vi "2 BoatInfotoStringSnapshot.vi"() -> (2 "Snapshot":string)   [LabVIEW 2011]
doc: "Makes a \"snapshot\" of robot status in string form, to be recorded in the log. Only notes what has changed since the last time."
uses:
  2 Classes/Waypoint/Waypoint.lvclass
  2 Globals/2 Global.vi
  Helper - Clean UTM Data.vi
  Helper - Clean Int Data.vi
  Helper - Clean String Data.vi
  Helper - Clean NoSail Data.vi
  Helper - Clean Boolean Data.vi
panel:
  in  "Array":string[](array[string])=["RobotLocation", "RobotHeading", "RobotVelocity", "RobotPitch", "RobotRoll", "BatteryVoltage", "ApparentWindDirection", "ApparentWindSpeed", "Rudder", "Sail", "GoodnessFunctions", "NoSailZones", "Waypoint#", "WaypointTolerance", "WaypointCoordinates", "OverrideRudder", "OverrideSail"]
  # "change this array if you want to record more things"
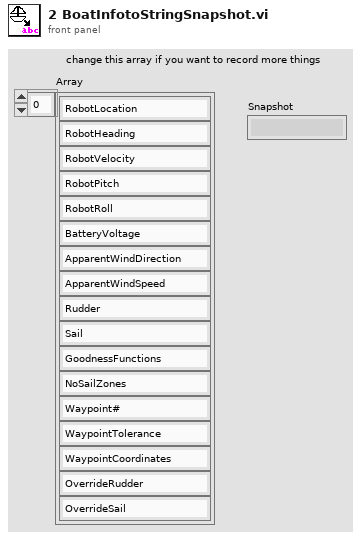
[diagram p1: front panel]
types:
  T1 = typedef "UTM Location.ctl" = cluster{"UTM Zone":dbl, "Hemisphere":enum16{"North", "South"}, "East":dbl, "North":dbl}
  T2 = typedef "heading.ctl" = dbl
  T3 = typedef "robot velocity.ctl" = cluster{"East":dbl, "North":dbl}
  T4 = typedef "pitch and roll.ctl" = cluster{"Pitch":dbl, "Roll":dbl}
  T5 = typedef "absolute wind direction.ctl" = dbl
  T6 = typedef "apparent wind speed.ctl" = dbl
  T7 = typedef "setpoints to boat.ctl" = cluster{"Sail Position":T8, "Rudder Angle":T9}
  T8 = typedef "sail setpt.ctl" = dbl
  T9 = typedef "rudder angle.ctl" = dbl
  T10 = typedef "Goodness Fns Indicator.ctl" = cluster{dbl, dbl, dbl[][]}
  T11 = typedef "UTM Circle.ctl" = cluster{"UTM Zone":dbl, "Hemisphere":enum16{"North", "South"}, "East":dbl, "North":dbl, "Radius":dbl}
  T12 = typedef "Current Waypoint.ctl" = i32
  T13 = typedef "Waypoints List.ctl" = refnum<class "Waypoint.lvclass">[]
  T14 = typedef "manual override.ctl" = cluster{"Override Active Rudder":bool, "Setpoints":T7, "Override Active Sail":bool}
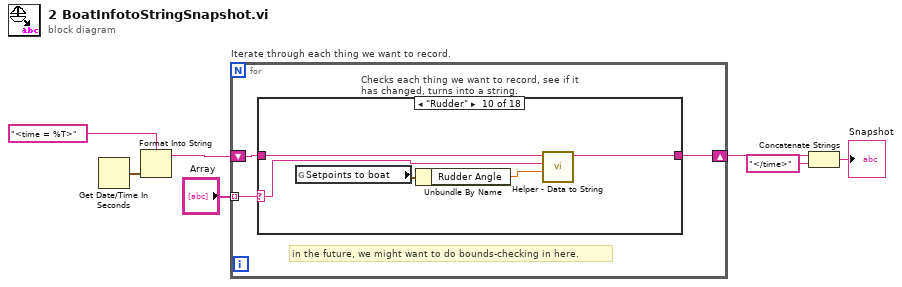
[diagram p0: block diagram]
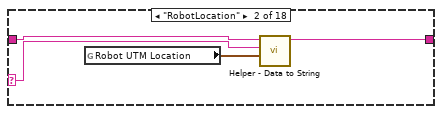
[diagram p3: hidden frame]
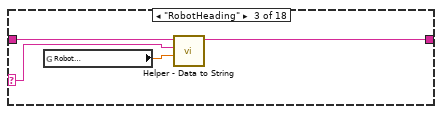
[diagram p4: hidden frame]
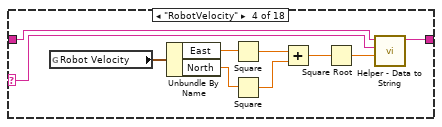
[diagram p5: hidden frame]
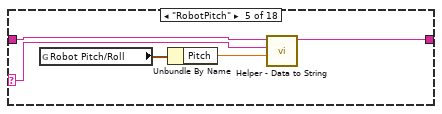
[diagram p6: hidden frame]
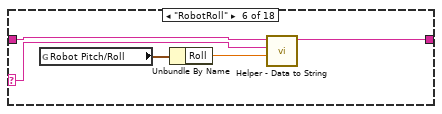
[diagram p7: hidden frame]
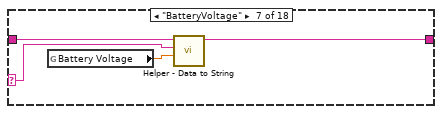
[diagram p8: hidden frame]
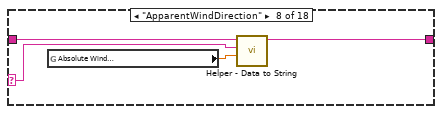
[diagram p9: hidden frame]
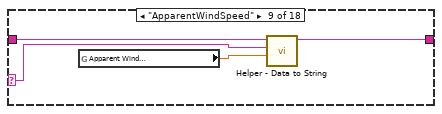
[diagram p10: hidden frame]
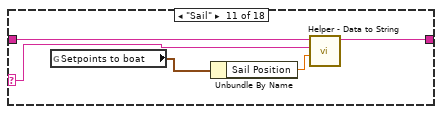
[diagram p11: hidden frame]
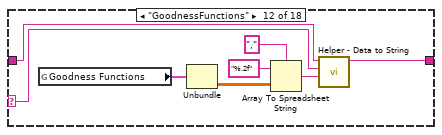
[diagram p12: hidden frame]
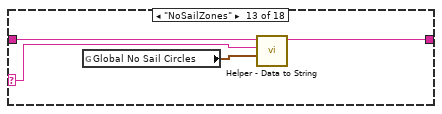
[diagram p13: hidden frame]
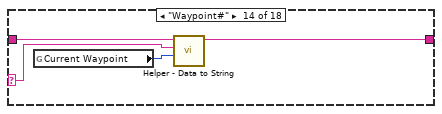
[diagram p14: hidden frame]
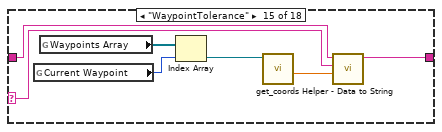
[diagram p15: hidden frame]
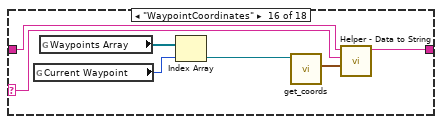
[diagram p16: hidden frame]
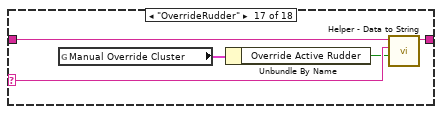
[diagram p17: hidden frame]
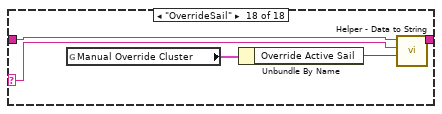
[diagram p18: hidden frame]
diagram:
  n1 = Get Date/Time In Seconds() -> (seconds since 1Jan1904=w7:timestamp)
  n2 = Format Into String(format string="<time = %T>" ("initial string"), w7) -> (resulting string=w4:string)  [unwired: 2 in, 1 out]
  n3 = for "Iterate through each thing we want to record." {
    tunnel: "Array" -> [w10] mode=indexing
    shift-right: [w9] -> w3
    shift-left: w4 -> [w8]
    # "in the future, we might want to do bounds-checking in here."
    n4 = case "Checks each thing we want to record, see if it has changed, turns into a string." shown="\"Rudder\"" w10 {
      selector: w10 -> [_ w12 w17 w27 w30 w35 w40 w44 w48 w54 w59 w67 w70 w74 w82 w86 w93 w97]
      tunnel: [w11 w14 w19 w29 w32 w37 w42 w46 w50 w56 w61 w69 w72 w76 w84 w85 w95 w99] -> w9
      tunnel: w8 -> [w11 w13 w16 w28 w31 w36 w41 w45 w49 w55 w60 w68 w71 w75 w83 w87 w94 w98]
      frame Default {
        # "hopefully never needs to be used"
      }
      frame "RobotLocation" {
        n5 = global read "2 Global.vi" "Robot UTM Location"() -> (w15:T1)
        n6 = call-poly "Helper - Data to String.vi"("Input"=w15, "Selector"=w12, "PrevString"=w13) -> ("Output"=w14:string)  [unwired: 8 in]
      }
      frame "RobotHeading" {
        n7 = global read "2 Global.vi" "Robot\nHeading"() -> (w18:T2)
        n8 = call-poly "Helper - Data to String.vi"("Input"=w18, "Selector"=w17, "PrevString"=w16) -> ("Output"=w19:string)  [unwired: 8 in]
      }
      frame "RobotVelocity" {
        n9 = global read "2 Global.vi" "Robot Velocity"() -> (w26:T3)
        n10 = Unbundle By Name(w26) -> ("East"=w25:dbl, "North"=w24:dbl)
        n11 = Square(x=w25) -> (x^2=w22:dbl)
        n12 = Square(x=w24) -> (x^2=w23:dbl)
        n13 = Add(x=w22, y=w23) -> (x+y=w21:dbl)
        n14 = Square Root(x=w21) -> (sqrt(x)=w20:dbl)
        n15 = call-poly "Helper - Data to String.vi"("Input"=w20, "Selector"=w27, "PrevString"=w28) -> ("Output"=w29:string)  [unwired: 8 in]
      }
      frame "RobotPitch" {
        n16 = global read "2 Global.vi" "Robot Pitch/Roll"() -> (w33:T4)
        n17 = Unbundle By Name(w33) -> ("Pitch"=w34:dbl)
        n18 = call-poly "Helper - Data to String.vi"("Input"=w34, "Selector"=w30, "PrevString"=w31) -> ("Output"=w32:string)  [unwired: 8 in]
      }
      frame "RobotRoll" {
        n19 = global read "2 Global.vi" "Robot Pitch/Roll"() -> (w38:T4)
        n20 = Unbundle By Name(w38) -> ("Roll"=w39:dbl)
        n21 = call-poly "Helper - Data to String.vi"("Input"=w39, "Selector"=w35, "PrevString"=w36) -> ("Output"=w37:string)  [unwired: 8 in]
      }
      frame "BatteryVoltage" {
        n22 = global read "2 Global.vi" "Battery Voltage"() -> (w43:dbl)
        n23 = call-poly "Helper - Data to String.vi"("Input"=w43, "Selector"=w40, "PrevString"=w41) -> ("Output"=w42:string)  [unwired: 8 in]
      }
      frame "ApparentWindDirection" {
        n24 = global read "2 Global.vi" "Absolute Wind\nDirection (º)"() -> (w47:T5)
        n25 = call-poly "Helper - Data to String.vi"("Input"=w47, "Selector"=w44, "PrevString"=w45) -> ("Output"=w46:string)  [unwired: 8 in]
      }
      frame "ApparentWindSpeed" {
        n26 = global read "2 Global.vi" "Apparent Wind\nSpeed"() -> (w51:T6)
        n27 = call-poly "Helper - Data to String.vi"("Input"=w51, "Selector"=w48, "PrevString"=w49) -> ("Output"=w50:string)  [unwired: 8 in]
      }
      frame "Rudder" {
        n28 = global read "2 Global.vi" "Setpoints to boat"() -> (w53:T7)
        n29 = Unbundle By Name(w53) -> ("Rudder Angle"=w52:T9)
        n30 = call-poly "Helper - Data to String.vi"("Input"=w52, "Selector"=w54, "PrevString"=w55) -> ("Output"=w56:string)  [unwired: 8 in]
      }
      frame "Sail" {
        n31 = global read "2 Global.vi" "Setpoints to boat"() -> (w58:T7)
        n32 = Unbundle By Name(w58) -> ("Sail Position"=w57:T8)
        n33 = call-poly "Helper - Data to String.vi"("Input"=w57, "Selector"=w59, "PrevString"=w60) -> ("Output"=w61:string)  [unwired: 8 in]
      }
      frame "GoodnessFunctions" {
        n34 = global read "2 Global.vi" "Goodness Functions"() -> (w64:T10)
        n35 = Unbundle(w64) -> (w66:dbl[][])  [unwired: 2 out]
        n36 = Array To Spreadsheet String(delimiter (Tab)=",", array=w66, 3:"%.2f" ("format string")) -> (spreadsheet string=w62:string)
        n37 = call-poly "Helper - Data to String.vi"("Input"=w62, "Selector"=w67, "PrevString"=w68) -> ("Output"=w69:string)  [unwired: 8 in]
      }
      frame "NoSailZones" {
        n38 = global read "2 Global.vi" "Global No Sail Circles"() -> (w73:T11[])
        n39 = call-poly "Helper - Data to String.vi"("Global No Sail Circles"=w73, "Selector"=w70, "PrevString"=w71) -> ("Output"=w72:string)  [unwired: 8 in]
      }
      frame "Waypoint#" {
        n40 = global read "2 Global.vi" "Current Waypoint"() -> (w77:T12)
        n41 = call-poly "Helper - Data to String.vi"("Input"=w77, "Selector"=w74, "PrevString"=w75) -> ("Output"=w76:string)  [unwired: 8 in]
      }
      frame "WaypointTolerance" {
        n42 = global read "2 Global.vi" "Current Waypoint"() -> (w81:T12)
        n43 = global read "2 Global.vi" "Waypoints Array"() -> (w80:T13)
        n44 = Index Array(array=w80, index=w81) -> (element=w79:refnum<class "Waypoint.lvclass">)
        n45 = call-dynamic "get_coords.vi"("Waypoint in"=w79) -> ("Tolerance (meters?)"=w78:dbl)  [unwired: 7 in, 3 out]
        n46 = call-poly "Helper - Data to String.vi"("Input"=w78, "Selector"=w82, "PrevString"=w83) -> ("Output"=w84:string)  [unwired: 8 in]
      }
      frame "WaypointCoordinates" {
        n47 = global read "2 Global.vi" "Current Waypoint"() -> (w91:T12)
        n48 = global read "2 Global.vi" "Waypoints Array"() -> (w90:T13)
        n49 = Index Array(array=w90, index=w91) -> (element=w89:refnum<class "Waypoint.lvclass">)
        n50 = call-dynamic "get_coords.vi"("Waypoint in"=w89) -> ("Coords"=w88:T1)  [unwired: 7 in, 3 out]
        n51 = call-poly "Helper - Data to String.vi"("Input"=w88, "Selector"=w86, "PrevString"=w87) -> ("Output"=w85:string)  [unwired: 8 in]
      }
      frame "OverrideRudder" {
        n52 = global read "2 Global.vi" "Manual Override Cluster"() -> (w96:T14)
        n53 = Unbundle By Name(w96) -> ("Override Active Rudder"=w92:bool)
        n54 = call-poly "Helper - Data to String.vi"("Input"=w92, "Selector"=w93, "PrevString"=w94) -> ("Output"=w95:string)  [unwired: 8 in]
      }
      frame "OverrideSail" {
        n55 = global read "2 Global.vi" "Manual Override Cluster"() -> (w101:T14)
        n56 = Unbundle By Name(w101) -> ("Override Active Sail"=w100:bool)
        n57 = call-poly "Helper - Data to String.vi"("Input"=w100, "Selector"=w97, "PrevString"=w98) -> ("Output"=w99:string)  [unwired: 8 in]
      }
    }
  }
  n58 = Concatenate Strings(w3, "</time>" ("string")) -> (→"Snapshot":string)
